vi "Create Menu from Folder.vi"(7 "Allow Initialization of AutoMenu on Target(T)":bool=TRUE, 8 "error in (no error)":errorcluster, 11 "Target Folder":path=path "C:/Program Files (x86)/National Instruments/LabVIEW 2019/user.lib/_Tools/Tools.Application") -> (0 "error out":errorcluster)   [LabVIEW 2019, in "AutoMenuCreator.lvlib"]
doc: "Create Menu files for 'Target Folder' at 'Menu Sub-folder'. If no Sub-folder is set (\"_Menu\" is the default value) no sub-folder will be used.\n\nNote:\nThe sub-folder will be deleted and re-created!"
uses:
  AutoMenuCreator.lvlib
  Ctl/Ctl_Run Data.ctl
  Ctl/Ctl_Config.ctl
  Ctl/Ctl_Config_Main.ctl
  Ctl/Ctl_Config_File Filter.ctl
  Ctl/Ctl_Config_Folder Filter.ctl
  Ctl/Ctl_Config_File Name Edit.ctl
  Ctl/Ctl_Config_Folder Name Edit.ctl
  Ctl/Ctl_Config_Folder Icon Map.ctl
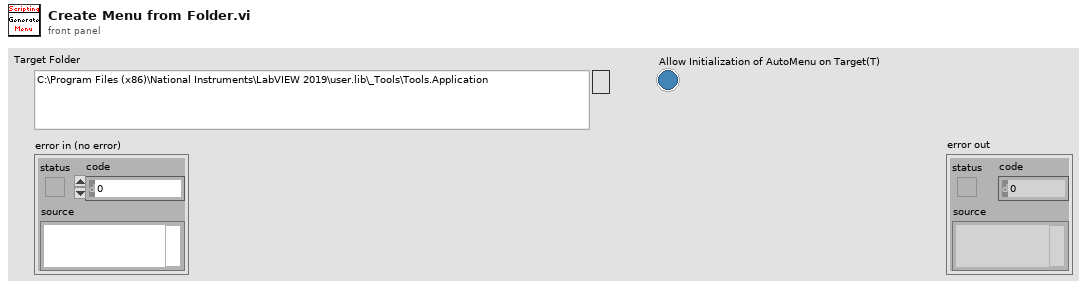
[diagram p1: front panel]
types:
  T1 = typedef "AutoMenuCreator.lvlib/Ctl_Run Data.ctl" = cluster{"Target Folder":path, "Menu Folder":path, "Active Folder":path, "Config":T2}
  T2 = typedef "AutoMenuCreator.lvlib/Ctl_Config.ctl" = cluster{"Main":T3, "File Filter":T4, "Folder Filter":T5, "File Name Edit":T6, "Folder Name Edit":T7, "Folder Icon Map":T8}
  T3 = typedef "AutoMenuCreator.lvlib/Ctl_Config_Main.ctl" = cluster{"Menu Folder":string, "Re-Create Menu Folder?":bool, "Allow mnu replace?":bool}
  T4 = typedef "AutoMenuCreator.lvlib/Ctl_Config_File Filter.ctl" = cluster{"Exclude Prefixes":string[], "Ignore Names":string[], "Include Extensions":string[], "Exclude Postfixes":string[]}
  T5 = typedef "AutoMenuCreator.lvlib/Ctl_Config_Folder Filter.ctl" = cluster{"Exclude Prefixes":string[], "Ignore Names":string[]}
  T6 = typedef "AutoMenuCreator.lvlib/Ctl_Config_File Name Edit.ctl" = cluster{"Pre Split String":string, "Post Split String":string}
  T7 = typedef "AutoMenuCreator.lvlib/Ctl_Config_Folder Name Edit.ctl" = cluster{"Pre Split String":string, "Post Split String":string, "Deletion Strings":string[]}
  T8 = typedef "AutoMenuCreator.lvlib/Ctl_Config_Folder Icon Map.ctl" = map{string, path}
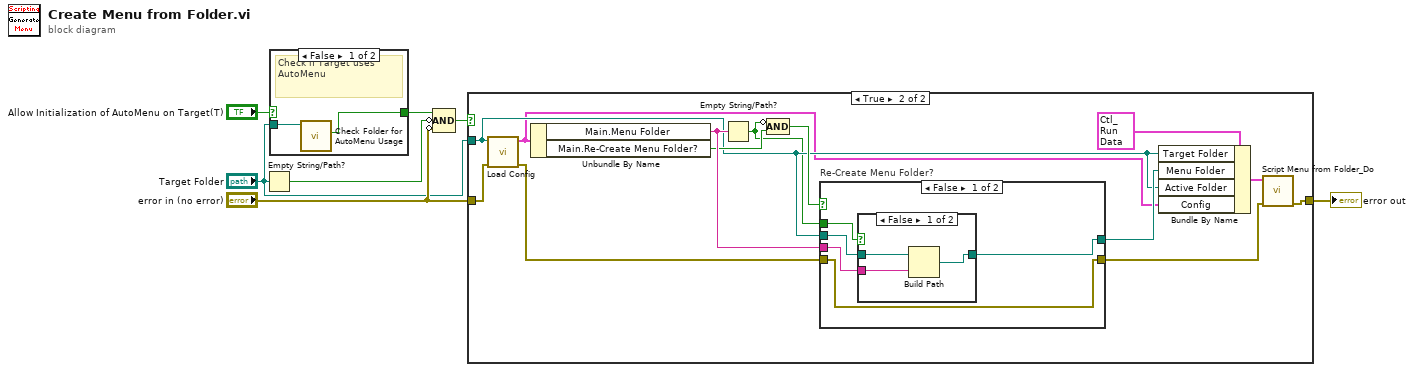
[diagram p0: block diagram]
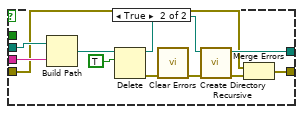
[diagram p5: hidden frame]
diagram:
  n1 = Empty String/Path?(string/path="Target Folder") -> (empty?=w6:bool)
  n2 = case shown="False" "Allow Initialization of AutoMenu on Target(T)" {
    selector: "Allow Initialization of AutoMenu on Target(T)" -> [_ w10]
    tunnel: "Target Folder" -> [w9 _]
    tunnel: [w8 w10] -> w1
    frame False {
      # "Check if Target uses  AutoMenu"
      n3 = call "Check Folder for AutoMenu Usage.vi"("Target Folder"=w9) -> ("Uses AutoMenu?"=w8:bool)  [unwired: 9 in, 1 out]
    }
    frame True {
      # "No check as init is allowed"
    }
  }
  n4 = Compound Arithmetic op=AND(w1, invert w6, invert "error in (no error)") -> (w4:bool)
  n5 = case shown="True" w4 {
    tunnel: "Target Folder" -> [_ w15]
    tunnel: [w11 w24] -> w7
    tunnel: "error in (no error)" -> [w11 w22]
    frame False {
    }
    frame True {
      n6 = call "Load Config.vi"("error in (no error)"=w22, "Target Folder"=w15) -> ("error out"=w18:errorcluster, "Config"=w14:T2)  [unwired: 8 in]
      n7 = Unbundle By Name(w14) -> ("Main.Menu Folder"=w21:string, "Main.Re-Create Menu Folder?"=w19:bool)
      n8 = Empty String/Path?(string/path=w21) -> (empty?=w12:bool)
      n9 = Compound Arithmetic op=AND(invert w12, w19) -> (w20:bool)
      n10 = case "Re-Create Menu Folder?" shown="False" w20 {
        tunnel: w18 -> [w29 w34]
        tunnel: [w29 w35] -> w23
        tunnel: [w27 w39] -> w16
        tunnel: w15 -> [w26 w38]
        tunnel: w21 -> [w25 w36]
        tunnel: w12 -> [w28 _]
        frame False {
          n11 = case shown="False" w28 {
            tunnel: [w31 w33] -> w27
            tunnel: w26 -> [w32 w33]
            tunnel: w25 -> [w30 _]
            frame False {
              n12 = Build Path(base path=w32, name or relative path=w30) -> (appended path=w31:path)
            }
            frame True {
            }
          }
        }
        frame True {
          n13 = Build Path(base path=w38, name or relative path=w36) -> (appended path=w37:path)
          n14 = Delete(path (use dialog)=w37, entire hierarchy (F)=TRUE) -> (deleted path=w43:path, error out=w42:errorcluster)  [unwired: 3 in, 1 out]
          n15 = call <vilib>:"Clear Errors.vi"("error in (no error)"=w42) -> ("error out"=w41:errorcluster)  [unwired: 5 in, 1 out]
          n16 = call <vilib>:"Create Directory Recursive.vi"("error in (no error)"=w41, "directory"=w43) -> ("error out"=w40:errorcluster, "directory copy"=w39:path)  [unwired: 3 in, 1 out]
          n17 = Merge Errors(w34, w40) -> (w35:errorcluster)
        }
      }
      n18 = Bundle By Name(cluster=T1 {"Target Folder"=path "", "Menu Folder"=path "", "Active Folder"=path "", "Config"={"Main"={"Menu Folder"="", "Re-Create Menu Folder?"=FALSE, "Allow mnu replace?"=FALSE}, "File Filter"={"Exclude Prefixes"=[], "Ignore Names"=[], "Include Extensions"=[], "Exclude Postfixes"=[]}, "Folder Filter"={"Exclude Prefixes"=[], "Ignore Names"=[]}, "File Name Edit"={"Pre Split String"="", "Post Split String"=""}, "Folder Name Edit"={"Pre Split String"="", "Post Split String"="", "Deletion Strings"=[]}, "Folder Icon Map"={}}} ("Run Data Cluster"), "Target Folder"=w15, "Menu Folder"=w16, "Active Folder"=w15, "Config"=w14) -> (w13:T1)
      n19 = call "Script Menu from Folder_Do.vi"("error in (no error)"=w23, "Run Data"=w13) -> ("error out"=w24:errorcluster)  [unwired: 8 in, 1 out]
    }
  }
  "error out" <- w7
